vi "Error Handler - Load Calibration.vi"(8 "error in":errorcluster) -> (0 "error out":errorcluster)   [LabVIEW 2021]
doc: "If an error is encountered loading calibration data, downgrade the error to a warning and continue."
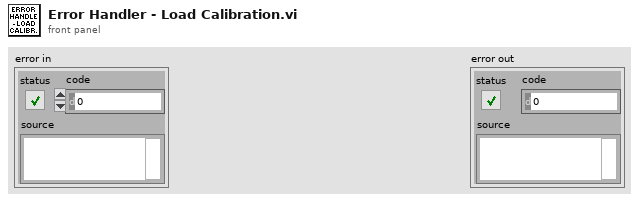
[diagram p1: front panel]
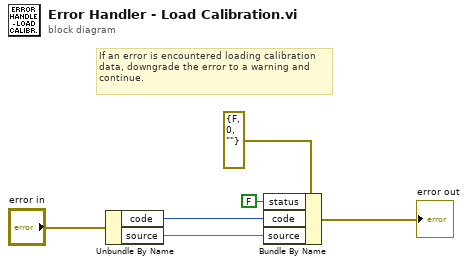
[diagram p0: block diagram]
diagram:
  # "If an error is encountered loading calibration\ndata, downgrade the error to a warning and\ncontinue."
  n1 = Unbundle By Name("error in") -> ("code"=w5:i32, "source"=w6:string)
  n2 = Bundle By Name(cluster=errorcluster {"status"=FALSE, "code"=0, "source"=""} ("error constant"), "status"=FALSE, "code"=w5, "source"=w6) -> (→"error out":errorcluster)
